vi "S7_WriteBools.vi"(7 "address":string, 8 "错误输入":errorcluster caption="错误输入（无错误）", 9 "values":bool[](array[boolean]), 11 "connect id":refnum<k24>) -> (0 "错误输出":errorcluster, 1 "values":bool[](array[boolean]), 2 "IsSuccess":bool, 3 "connect id":refnum<k24>)   [LabVIEW 2018]
uses:
  E:/Fergus/S7/S7_code/Lib/HslCommunication.dll
  Lib/HslCommunication.dll
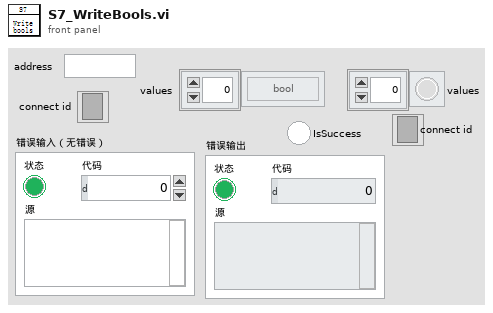
[diagram p1: front panel]
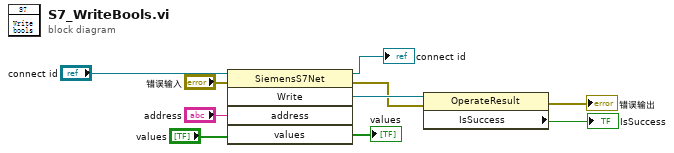
[diagram p0: block diagram]
diagram:
  n1 = invoke on="调用节点" class="SiemensS7Net" method="Write"(reference="connect id", error in="错误输入", "address"="address", "values"="values") -> (reference out=→"connect id":refnum<k24>, error out=w5:errorcluster, "Write"=w7:refnum<k24>, "values"=→"values":bool[])  [unwired: 1 in, 1 out]
  n2 = property class="OperateResult"(reference=w7, error in=w5) -> (error out=→"错误输出":errorcluster, "IsSuccess"=→"IsSuccess":bool)  [unwired: 1 out]
